vi "UTC_time.vi"() -> ()   [LabVIEW 2019]
uses:
  <vilib>/Utility/miscctls.llb/LVDateTimeRec.ctl
panel:
  out "unsigned 64bit integer 2":u64
  out "UTC Timestamp":u64
  in  "date time rec 2":T1
  out "double precision float":dbl
  out "time stamp 2":timestamp
  in  "number":dbl
  out "unsigned 64bit integer":u64
  out "time stamp":timestamp
  out "date time rec":T1
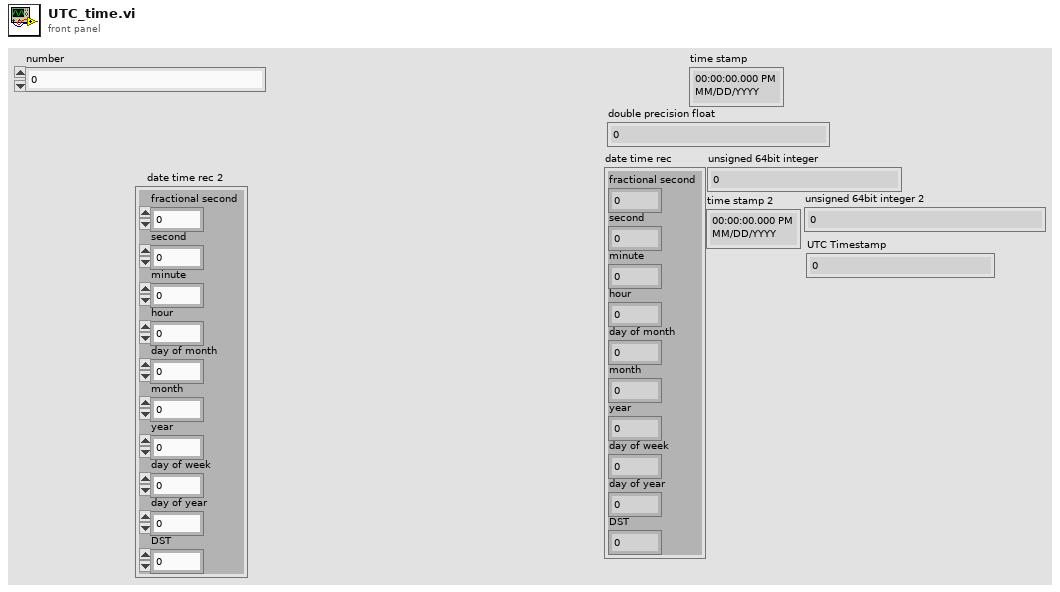
[diagram p1: front panel]
types:
  T1 = typedef "LVDateTimeRec.ctl" = cluster{"fractional second":dbl, "second":i32, "minute":i32, "hour":i32, "day of month":i32, "month":i32, "year":i32, "day of week":i32, "day of year":i32, "DST":i32}
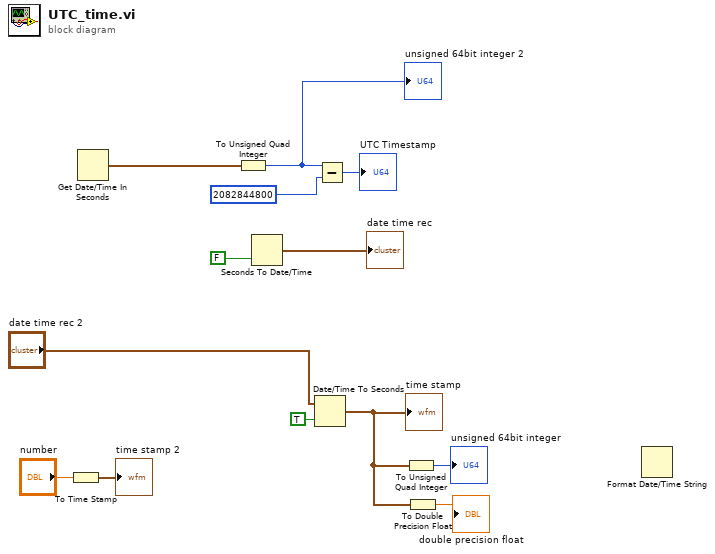
[diagram p0: block diagram]
diagram:
  n1 = To Time Stamp(1:"number") -> (0:→"time stamp 2":timestamp)
  n2 = Get Date/Time In Seconds() -> (seconds since 1Jan1904=w4:timestamp)
  n3 = To Unsigned Quad Integer(1:w4) -> (0:w1:u64)
  "unsigned 64bit integer 2" <- w1
  n4 = Seconds To Date/Time(to UTC (F)=FALSE) -> (date time rec=→"date time rec":T1)  [unwired: 1 in]
  n5 = Date/Time To Seconds(1:TRUE ("is UTC (F)"), 2:"date time rec 2") -> (0:w8:timestamp)
  "time stamp" <- w8
  n6 = Subtract(x=w1, y=u64 2082844800) -> (x-y=→"UTC Timestamp":u64)
  n7 = To Unsigned Quad Integer(1:w8) -> (0:→"unsigned 64bit integer":u64)
  n8 = To Double Precision Float(number=w8) -> (double precision float=→"double precision float":dbl)
  n9 = Format Date/Time String() -> ()  [unwired: 3 in, 1 out]
